vi "I2C.vi"() -> ()   [LabVIEW 2019]
uses:
  <vilib>/myRIO/Instrument Drivers/Onboard IO/I2C/typedefs/I2C User Configuration.ctl
  <vilib>/myRIO/Instrument Drivers/Onboard IO/I2C/typedefs/I2C Transfer Rate.ctl
  <vilib>/myRIO/Instrument Drivers/Onboard IO/I2C/typedefs/I2C Reference.ctl
  <vilib>/myRIO/Common/Instrument Driver Framework/Utilities/typedefs/myRIO Generic Hardware Reference.ctl
  <vilib>/myRIO/Common/Instrument Driver Framework/Utilities/typedefs/Hardware Version Enum.ctl
  <vilib>/myRIO/Common/Instrument Driver Framework/Utilities/typedefs/myRIO v1.0 Reference.ctl
  <vilib>/myRIO/Common/Instrument Driver Framework/Utilities/typedefs/Generic FPGA Reference.ctl
  <vilib>/myRIO/Common/Instrument Driver Framework/myRIO v1.0/I2C/typedefs/I2C Channels Enum.ctl
  <vilib>/myRIO/Instrument Drivers/Onboard IO/I2C/typedefs/I2C Configuration.ctl
  <vilib>/userdefined/High Color/nirio_resource_hc.ctl
  <vilib>/myRIO/Common/Instrument Driver Framework/Utilities/vis/Validate Channels.vi
  <vilib>/myRIO/Common/Instrument Driver Framework/myRIO v1.0/UART/vis/myRIO v1.0 Close UART.vi
  <vilib>/myRIO/Common/Instrument Driver Framework/ELVIS III v1.0/Resource Manager/vis/ELVIS III v1.0 Create Configuration List.vi
  <vilib>/Utility/VariantDataType/GetNumericInfo.vi
  <vilib>/Utility/error.llb/Error Cluster From Error Code.vi
  <vilib>/myRIO/Common/Instrument Driver Framework/ELVIS III v1.0/ELVIS III v1.1 Open.vi
  <vilib>/myRIO/Common/Instrument Driver Framework/ELVIS III v1.0/Resource Manager/vis/ELVIS III v1.0 Reserve Channel List.vi
  <vilib>/myRIO/Common/Instrument Driver Framework/ELVIS III v1.0/Resource Manager/vis/ELVIS III v1.0 Configure IO.vi
  <vilib>/myRIO/Common/Instrument Driver Framework/myRIO v1.0/myRIO v1.0 Close.vi
  <vilib>/myRIO/Common/Instrument Driver Framework/ELVIS III v1.0/Resource Manager/vis/ELVIS III v1.0 Unreserve Channel List.vi
  <vilib>/myRIO/Common/Instrument Driver Framework/Utilities/vis/FPGA Ref Manager.vi
  <vilib>/myRIO/Common/Instrument Driver Framework/ELVIS III v1.0/ELVIS III v1.0 Reset FPGA.vi
  <vilib>/myRIO/Common/Instrument Driver Framework/myRIO v1.0/IRQ/vis/myRIO v1.0 IRQ Info FGV.vi
  <vilib>/myRIO/Common/Instrument Driver Framework/myRIO v1.0/IRQ/vis/myRIO v1.0 Timer IRQ Info FGV.vi
  <vilib>/myRIO/Common/Instrument Driver Framework/myRIO v1.0/IRQ/vis/myRIO v1.0 ISR Agent.vi
  <vilib>/myRIO/Instrument Drivers/Utilities/vis/Reset Index.vi
  <vilib>/myRIO/Common/Instrument Driver Framework/myRIO v1.0/Resource Manager/vis/myRIO v1.0 Block Write Resource Manager.vi
  <vilib>/myRIO/Instrument Drivers/Onboard IO/I2C/vis/myRIO I2C Open.xnode
  <vilib>/myRIO/Instrument Drivers/Utilities/Utilities.lvlib
  <vilib>/myRIO/Instrument Drivers/Onboard IO/I2C/I2C.lvlib
panel:
  out "Acceleration Data":T1(graph)={"Decimal Number Out"=0.14069369809477283, "Decimal Number Out"=0.9848558866634098, "Decimal Number Out"=0.14069369809477283}
  in  "Stop":bool
  out "Raw data":u8[](array[numeric]) format="%x"
  in  "Slave Address (7-bit)":u8=29 format="%x"
  # "ELVIS III Control IO"
  # "I2C"
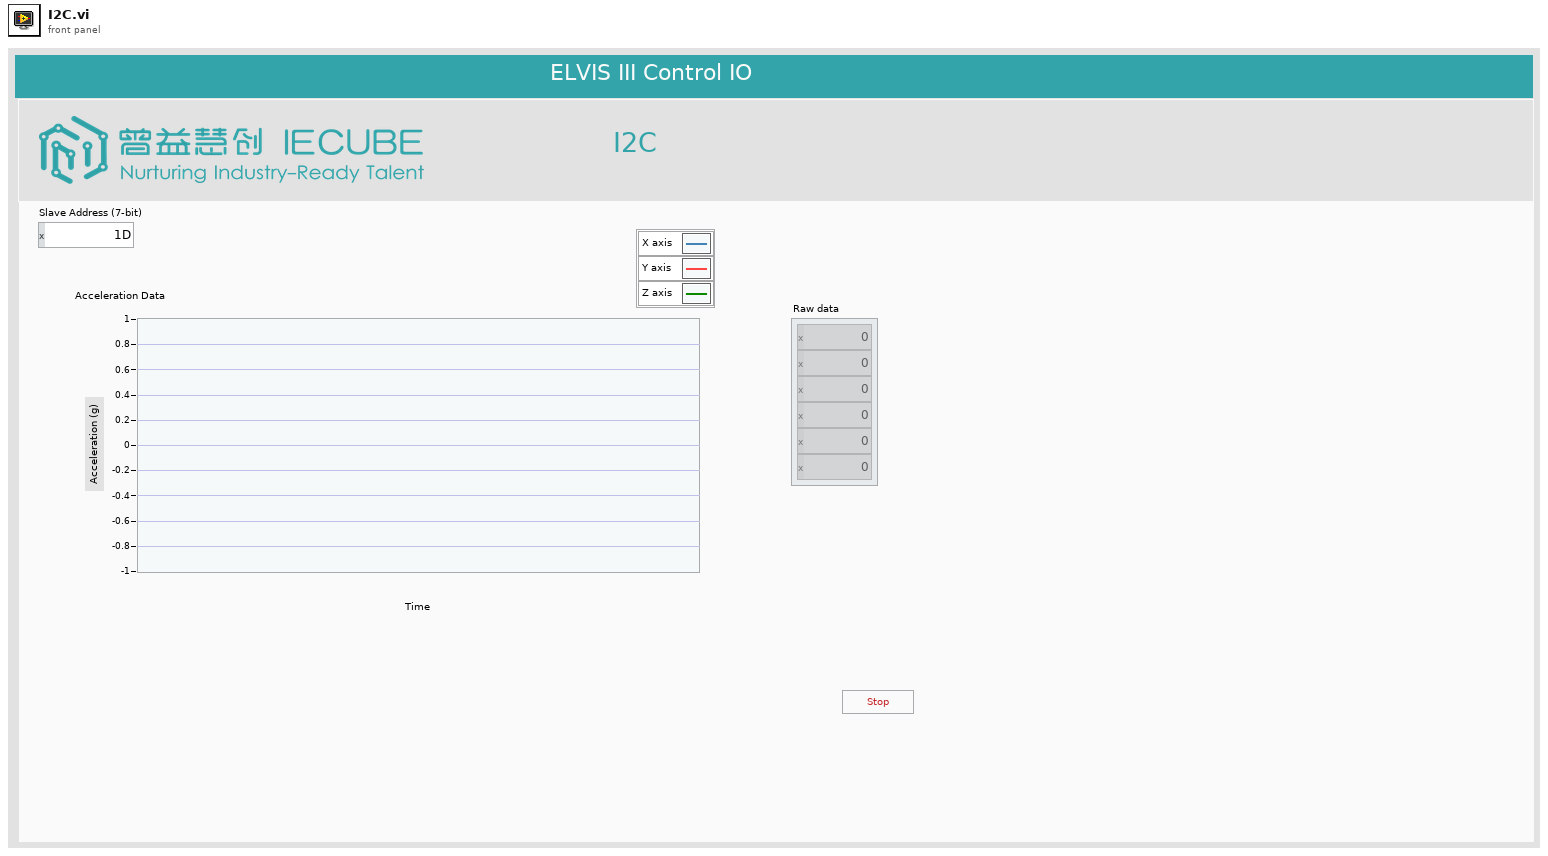
[diagram p1: front panel]
types:
  T1 = cluster{"Decimal Number Out":dbl, "Decimal Number Out":dbl, "Decimal Number Out":dbl}
  T2 = typedef "I2C.lvlib/I2C User Configuration.ctl" = cluster{"I2C Transfer Rate":T3}
  T3 = typedef "I2C.lvlib/I2C Transfer Rate.ctl" = enum16{"Standard mode (100 kbps)", "Fast mode (400 kbps)"}
  T4 = cluster{"Decimal Number Out":dbl, "Decimal Number Out":dbl, "Decimal Number Out":dbl}[]
  T5 = typedef "nirio_resource_hc.ctl" = tag
  T6 = typedef "Hardware Version Enum.ctl" = enum16{"Unknown", "myRIO-1900", "myRIO-1950", "roboRIO", "NI ELVIS RIO CM", "ELVIS III"}
  T7 = typedef "I2C.lvlib/I2C Reference.ctl" = cluster{"myRIO Reference":T8, "I2C Channels Enum":T11, "I2C Configuration":T12}
  T8 = typedef "myRIO Generic Hardware Reference.ctl" = cluster{"myRIO Model":T6, "myRIO Hardware Reference":T9}
  T9 = typedef "myRIO v1.0 Reference.ctl" = cluster{"Generic FPGA Reference":T10, "Allow multiple opens":bool}
  T10 = typedef "Generic FPGA Reference.ctl" = refnum<k20>
  T11 = typedef "I2C Channels Enum.ctl" = enum16{"Not Connected", "A/I2C", "B/I2C", "I2C/I2C"}
  T12 = typedef "I2C.lvlib/I2C Configuration.ctl" = cluster{"I2C Transfer Rate":T3}
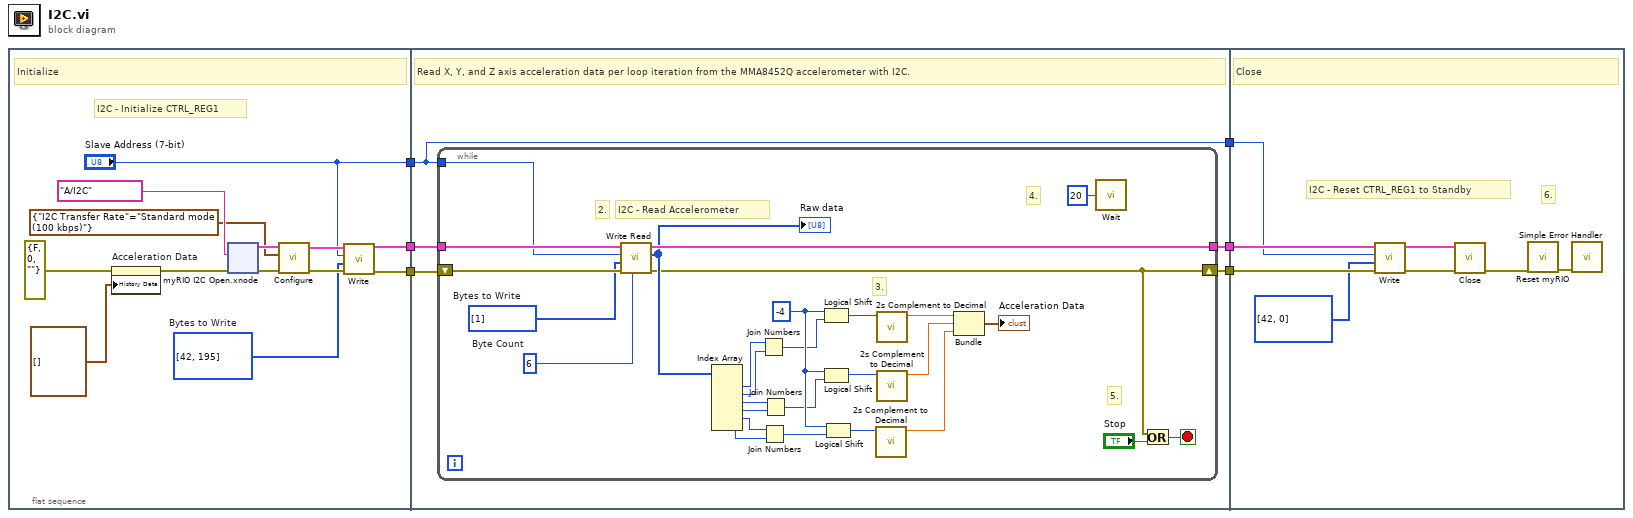
[diagram p0: block diagram]
diagram:
  n1 = flat-sequence {
    tunnel: ["Slave Address (7-bit)"] -> w5
    tunnel: [w8] -> w3
    tunnel: [w7] -> w2
    tunnel: [w40] -> w6
    tunnel: w5 -> [w39]
    tunnel: [w39] -> w4
    tunnel: w3 -> [w38]
    tunnel: w2 -> [w37]
    tunnel: [w36] -> w1
    tunnel: w6 -> [w75]
    tunnel: w4 -> [w73]
    tunnel: w1 -> [w74]
    frame #0 {
      w10 = u8[] [42, 195]  # Bytes to Write
      # "I2C - Initialize CTRL_REG1"
      # "Initialize"
      n2 = property on="Acceleration Data" class="WFChart (严格)"(error in=errorcluster {"status"=FALSE, "code"=0, "source"=""} ("Error In"), "History Data"=T4 []) -> (error out=w16:errorcluster)  [unwired: 1 in, 1 out]
      n3 = xnode "myRIO I2C Open.xnode"("error in (no error)"=w16, "Channel Name"=tag "A/I2C") -> ("error out"=w15:errorcluster, "I2C Ref Out"=w14:T7)  [unwired: 1 in]
      n4 = call <vilib>:"Configure.vi"("error in (no error)"=w15, "I2C User Configuration"=T2 {"I2C Transfer Rate"=enum."Standard mode (100 kbps)"}, "I2C Ref In"=w14) -> ("error out"=w12:errorcluster, "I2C Ref Out"=w11:T7)  [unwired: 7 in]
      n5 = call <vilib>:"Write.vi"("error in (no error)"=w12, "Bytes to Write"=w10, "Slave Address (7-bit)"="Slave Address (7-bit)", "I2C Ref In"=w11) -> ("error out"=w8:errorcluster, "I2C Ref Out"=w7:T7)  [unwired: 6 in]
    }
    frame #1 {
      # "Read X, Y, and Z axis acceleration data per loop iteration from the MMA8452Q accelerometer with I2C."
      n6 = while {
        shift-right: [w41] -> w40
        shift-left: w38 -> [w54]
        tunnel: w39 -> [w52]
        tunnel: w37 -> [w53]
        tunnel: [w49] -> w36
        stop <- w63 stop-if-true
        w50 = u32 6  # Byte Count
        w51 = u8[] [1]  # Bytes to Write
        w67 = i16 -4 ("y")
        # "I2C - Read Accelerometer"
        # "5."
        # "4."
        # "3."
        # "2."
        n7 = call <vilib>:"Write Read.vi"("Byte Count"=w50, "error in (no error)"=w54, "Bytes to Write"=w51, "Slave Address (7-bit)"=w52, "I2C Ref In"=w53) -> ("error out"=w41:errorcluster, "Bytes Read"=w48:u8[], "I2C Ref Out"=w49:T7)  [unwired: 3 in]
        "Raw data" <- w48
        n8 = Index Array(array=w48) -> (element #1=w47:u8, element #2=w46:u8, element #3=w45:u8, element #4=w44:u8, element #5=w43:u8, element #6=w42:u8)  [unwired: 6 in]
        n9 = Join Numbers(hi=w47, lo=w46) -> ((hi.lo)=w64:u16)
        n10 = Join Numbers(hi=w43, lo=w42) -> ((hi.lo)=w66:u16)
        n11 = Join Numbers(hi=w45, lo=w44) -> ((hi.lo)=w65:u16)
        n12 = Logical Shift(y=w67, x=w64) -> (x << y=w62:u16)
        n13 = Logical Shift(y=w67, x=w65) -> (x << y=w61:u16)
        n14 = Logical Shift(y=w67, x=w66) -> (x << y=w55:u16)
        n15 = call "2s Complement to Decimal.vi"("2s Complement In"=w55) -> ("Decimal Number Out"=w58:dbl)  [unwired: 10 in]
        n16 = call "2s Complement to Decimal.vi"("2s Complement In"=w62) -> ("Decimal Number Out"=w60:dbl)  [unwired: 10 in]
        n17 = call "2s Complement to Decimal.vi"("2s Complement In"=w61) -> ("Decimal Number Out"=w59:dbl)  [unwired: 10 in]
        n18 = Bundle("Decimal Number Out"=w60, "Decimal Number Out"=w59, "Decimal Number Out"=w58) -> (→"Acceleration Data":T1)  [unwired: 1 in]
        n19 = call "Wait"("Count(mSec)"=u32 20) -> ()  [unwired: 1 out]
        n20 = Or(x=w41, y="Stop") -> (x .or. y?=w63:bool)
      }
    }
    frame #2 {
      # "I2C - Reset CTRL_REG1 to Standby"
      # "6."
      # "Close"
      n21 = call <vilib>:"Write.vi"("error in (no error)"=w75, "Bytes to Write"=u8[] [42, 0], "Slave Address (7-bit)"=w73, "I2C Ref In"=w74) -> ("error out"=w71:errorcluster, "I2C Ref Out"=w70:T7)  [unwired: 6 in]
      n22 = call <vilib>:"Close.vi"("error in (no error)"=w71, "I2C Ref In"=w70) -> ("error out"=w69:errorcluster)  [unwired: 9 in]
      n23 = call <vilib>:"Reset myRIO.vi"("error in (no error)"=w69) -> ("error out"=w76:errorcluster)  [unwired: 10 in]
      n24 = call <vilib>:"Simple Error Handler.vi"("error in (no error)"=w76) -> ()  [unwired: 4 in, 5 out]
    }
  }
